vi "LOEM_Lv_Measurement.vi"(9 "Calibration Ch":i32(ring) items=["U00", "U01", "U02", "U03", "U04"], 10 "ManualMeasurementTime":dbl=0.1) -> (1 "Lv Display":dbl)   [LabVIEW 2019]
uses:
  C:/Program Files (x86)/National Instruments/LabVIEW 2019/LC-MISDK.dll
  Program Files (x86)/National Instruments/LabVIEW 2019/LC-MISDK.dll
panel:
  out "Lv":dbl
  out "error out":errorcluster
  # "Reprogramado Por Fredy Osorio 05/2025\ning.fredyosorio@gmail.com\nhttps://github.com/fr3dyos/PUC-LOEM-Controle-Minolta"
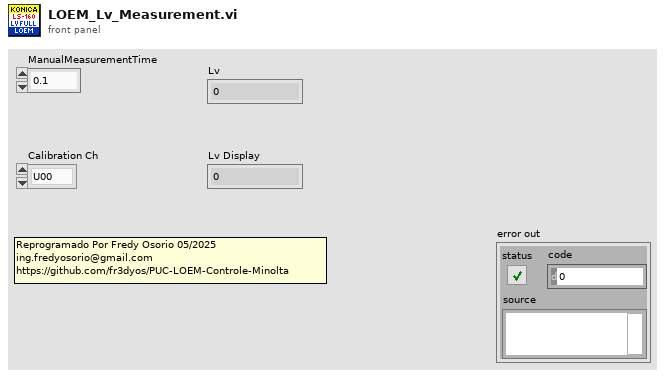
[diagram p1: front panel]
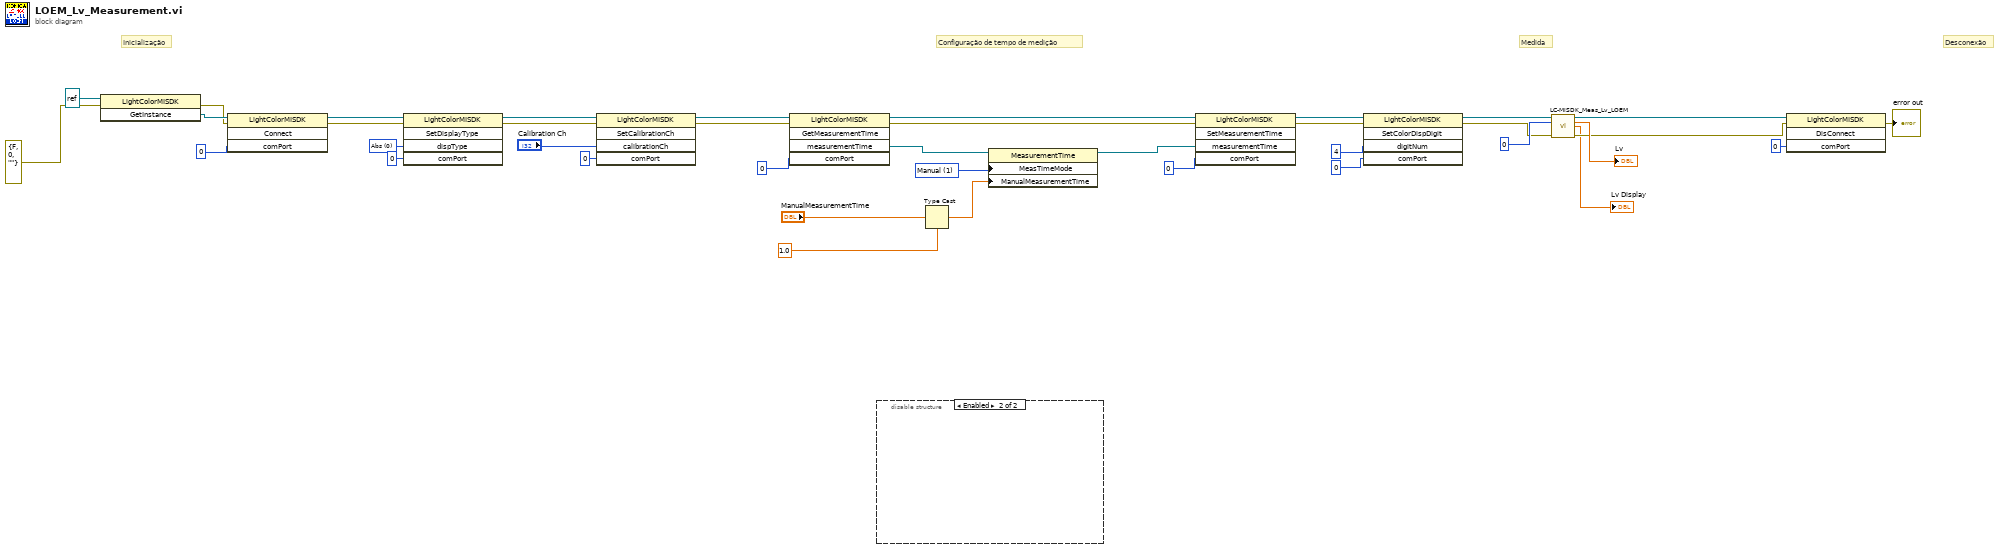
[diagram p0: block diagram]
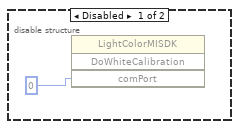
[diagram p2: hidden frame]
diagram:
  w20 = 0 items=["Abs", "Diff", "Ratio"] ("dispType")
  w35 = 1 items=["Auto", "Manual"] ("MeasTimeMode")
  # "Desconexão"
  # "Medida"
  # "Inicialização"
  # "Configuração de tempo de medição"
  n1 = invoke class="LightColorMISDK" method="GetInstance"(reference=refnum<k24> refnum, error in=errorcluster {"status"=FALSE, "code"=0, "source"=""} ("error in (no error)")) -> (error out=w14:errorcluster, "GetInstance"=w37:refnum<k24>)  [unwired: 1 in, 1 out]
  n2 = invoke class="LightColorMISDK" method="Connect"(reference=w37, error in=w14, "comPort"=0) -> (reference out=w22:refnum<k24>, error out=w13:errorcluster)  [unwired: 1 in, 2 out]
  n3 = invoke class="LightColorMISDK" method="SetDisplayType"(reference=w22, error in=w13, "dispType"=w20, "comPort"=0) -> (reference out=w19:refnum<k24>, error out=w12:errorcluster)  [unwired: 1 in, 3 out]
  n4 = invoke class="LightColorMISDK" method="SetCalibrationCh"(reference=w19, error in=w12, "calibrationCh"="Calibration Ch", "comPort"=0) -> (reference out=w18:refnum<k24>, error out=w11:errorcluster)  [unwired: 1 in, 3 out]
  n5 = invoke class="LightColorMISDK" method="GetMeasurementTime"(reference=w18, error in=w11, "comPort"=0) -> (reference out=w32:refnum<k24>, error out=w10:errorcluster, "measurementTime"=w31:refnum<k24>)  [unwired: 2 in, 2 out]
  n6 = disable-structure shown="Enabled" {
    frame Disabled {
      n7 = invoke class="LightColorMISDK" method="DoWhiteCalibration"("comPort"=0 ("DoWhiteCalibration")) -> ()  [unwired: 3 in, 4 out]
    }
    frame Enabled {
    }
  }
  n8 = Type Cast(type=1.0, x="ManualMeasurementTime") -> (*(type *) &x=w23:dbl)
  n9 = property class="MeasurementTime"(reference=w31, "MeasTimeMode"=w35, "ManualMeasurementTime"=w23) -> (reference out=w34:refnum<k24>)  [unwired: 1 in, 1 out]
  n10 = invoke class="LightColorMISDK" method="SetMeasurementTime"(reference=w32, error in=w10, "measurementTime"=w34, "comPort"=0) -> (reference out=w26:refnum<k24>, error out=w9:errorcluster)  [unwired: 1 in, 3 out]
  n11 = invoke class="LightColorMISDK" method="SetColorDispDigit"(reference=w26, error in=w9, "digitNum"=i16 4, "comPort"=0) -> (reference out=w2:refnum<k24>, error out=w1:errorcluster)  [unwired: 1 in, 3 out]
  n12 = call "LC-MISDK_Meas_Lv_LOEM.vi"(".NET reference"=w2, "comPort"=0, "error in"=w1) -> (".NET reference out"=w5:refnum<k24>, "Lv"=→"Lv":dbl, "Lv Display"=→"Lv Display":dbl, "error out"=w4:errorcluster)  [unwired: 8 in, 1 out]
  n13 = invoke on="インボークノード" class="LightColorMISDK" method="DisConnect"(reference=w5, error in=w4, "comPort"=0) -> (error out=→"error out":errorcluster)  [unwired: 1 in, 3 out]
